vi "VI Server_RUN VI.vi"(6 "Wait Until Done":bool, 8 "Error In":errorcluster, 11 "VI Path":path) -> (0 "Error out":errorcluster)   [LabVIEW 2020, in "VI Server Toolkit LV2013.lvlib"]
doc: "Programmatically runs targeted VI.\nCan be used in a debugging process."
uses:
  VI Server Toolkit LV2013.lvlib
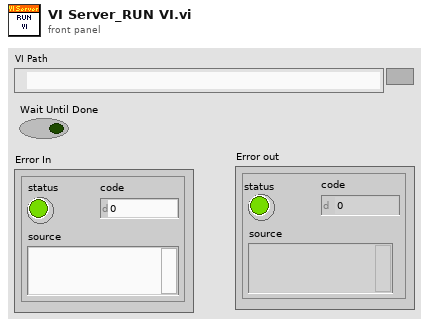
[diagram p1: front panel]
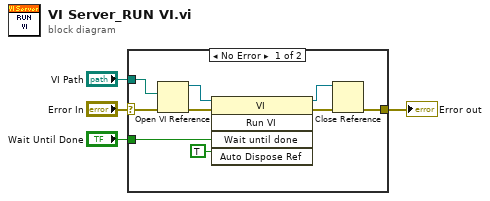
[diagram p0: block diagram]
diagram:
  n1 = case shown="No Error" "Error In" {
    selector: "Error In" -> [w5 w14]
    tunnel: "VI Path" -> [w13 _]
    tunnel: "Wait Until Done" -> [w10 _]
    tunnel: [w6 w14] -> w2
    frame No Error {
      n2 = Open VI Reference(vi path=w13, error in (no error)=w5) -> (vi reference=w11:refnum<vi>, error out=w12:errorcluster)  [unwired: 4 in]
      n3 = invoke class="VI" method="Run VI"(reference=w11, error in=w12, "Wait until done"=w10, "Auto Dispose Ref"=TRUE ("Auto Dispose Reference")) -> (reference out=w7:refnum<vi>, error out=w8:errorcluster)  [unwired: 1 in, 3 out]
      n4 = Close Reference(reference=w7, error in (no error)=w8) -> (error out=w6:errorcluster)
    }
    frame Error {
    }
  }
  "Error out" <- w2
